vi "Client.vi"() -> ()   [LabVIEW 2015]
uses:
  <vilib>/imath/engines/lvmath2/RunTimeEngine/Managers/WorkSpace/UID Generator.vi
  <vilib>/imath/engines/lvmath/Plug In/Control Design/BuiltInFunctions/tf/NIMS_CD_tf(STR,Ts).vi
  <vilib>/imathl/engines/lvmath/Functions/Error Handling/Create Error.vi
  <vilib>/imath/engines/lvmath/Plug In/Control Design/BuiltInFunctions/multmx/NIMS_CD_multmx(TF,K).vi
  <vilib>/imath/engines/lvmath/Plug In/Control Design/BuiltInFunctions/plus/NIMS_CD_plus(K,TF).vi
  <vilib>/imath/engines/lvmath/Functions/Error Handling/MergeErrorsWrapper.vi
  <vilib>/imath/engines/lvmath/Plug In/Control Design/BuiltInFunctions/powermx/NIMS_CD_powermx(TF,N).vi
  <vilib>/imath/engines/lvmath/Plug In/Control Design/BuiltInFunctions/plus/NIMS_CD_plus(TF,TF).vi
  <vilib>/imath/engines/lvmath/Plug In/Control Design/BuiltInFunctions/rightdivmx/NIMS_CD_rightdivmx(TF,TF).vi
  <vilib>/imath/engines/lvmath2/RunTimeEngine/RunTimeType/NIMS_RunTimeType_From StrictType (excl LVString).vi
  <instcachedir>/0/NIMS_RunTimeType_From StrictType (excl LVString)_EB1C38A9BC5048DA9ABDA8F781E54D21.lvgen/NIMS_RunTimeType_From StrictType (excl LVString)_EB1C38A9BC5048DA9ABDA8F781E54D21_031.vi
  <vilib>/imath/engines/lvmath2/RunTimeEngine/LocalVariableDefStatement/MC_LocalVariableDefStatement_Display.vi
  <vilib>/imath/engines/lvmath/Plug In/Control Design/BuiltInFunctions/multmx/NIMS_CD_multmx(K,TF).vi
  <vilib>/imath/engines/lvmath/Plug In/Control Design/BuiltInFunctions/rightdivmx/NIMS_CD_rightdivmx(TF,K).vi
  <vilib>/imath/engines/lvmath/Plug In/Control Design/BuiltInFunctions/step/NIMS_CD_[Y,T]=step(TF,[Tinfo]).vi
  <vilib>/imath/engines/lvmath2/RunTimeEngine/Managers/SymbolTable/Clear UID.vi
  <vilib>/imath/engines/lvmath2/RunTimeEngine/NodeEndStatement/NIMS_NodeEndStatement_Output.vi
  <instcachedir>/0/NIMS_NodeEndStatement_Output_53EC0D466D134D7ABD903AC30B43404B.lvgen/NIMS_NodeEndStatement_Output_53EC0D466D134D7ABD903AC30B43404B_002.vi
  <vilib>/imath/engines/lvmath2/RunTimeEngine/ErrorHandling/NIMS_Finalize Error.vi
  <vilib>/imath/engines/lvmath2/RunTimeEngine/Managers/SymbolTable/NIMS_WorkSpace.lvlib
panel:
  out "JSON string":string
  in  "stop":bool
  out "error out":errorcluster
  in  "error in (no error)":errorcluster
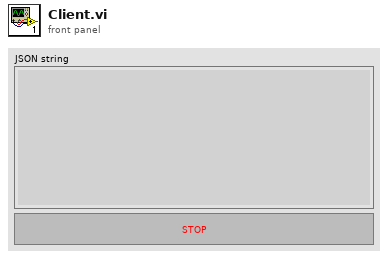
[diagram p1: front panel]
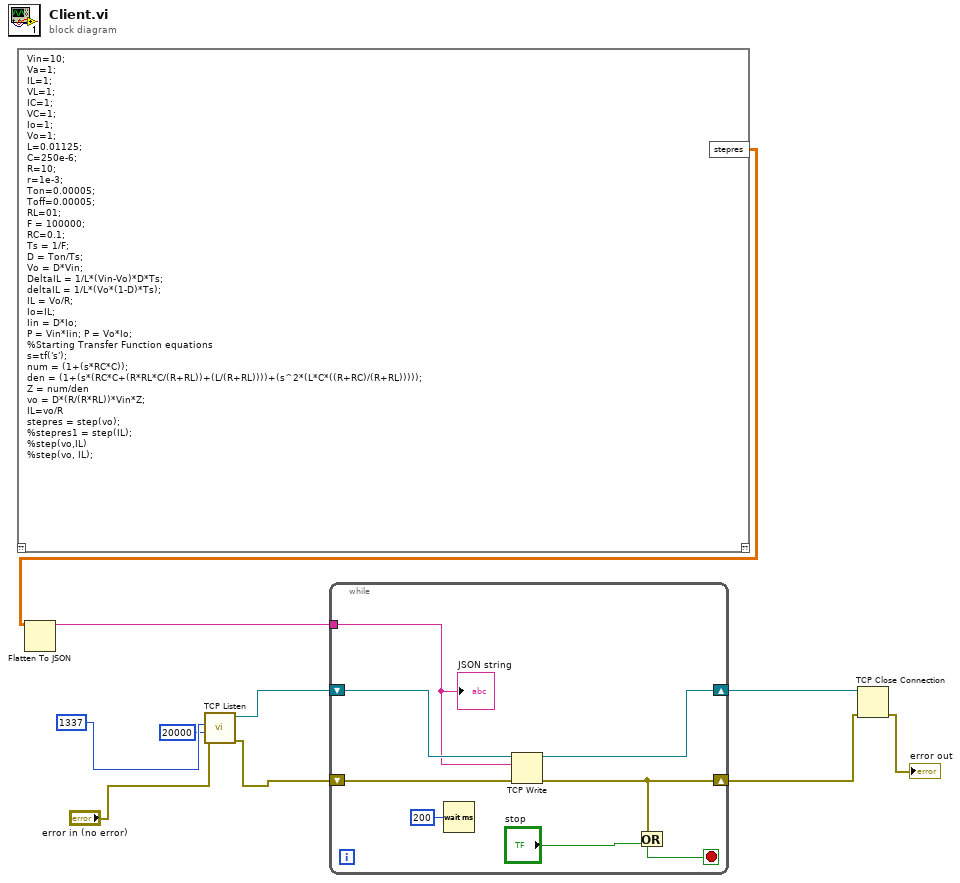
[diagram p0: block diagram]
diagram:
  n1 = mathscript code="Vin=10;\nVa=1;\nIL=1;\nVL=1;\nIC=1;\nVC=1;\nIo=1;\nVo=1;\nL=0.01125;\nC=250e-6;\nR=10;\nr=1e-3;\nTon=0.00005;\nToff=0.00005;\nRL=01;\nF = 100000;\nRC=0.1;\nTs = 1/F;\nD = Ton/Ts;\nVo = D*Vin;\nDeltaIL = 1/L*(Vin-Vo)*D*Ts;\ndeltaIL = 1/L*(Vo*(1-D)*Ts);\nIL = Vo/R;\nIo=IL;\nIin = D*Io;\nP = Vin*Iin; P = Vo*Io;\n%Starting Transfer Function equations\ns=tf('s');\nnum = (1+(s*RC*C));\nden = (1+(s*(RC*C+(R*RL*C/(R+RL))+(L/(R+RL))))+(s^2*(L*C*((R+RC)/(R+RL)))));\nZ = num/den\nvo = D*(R/(R*RL))*Vin*Z;\nIL=vo/R\nstepres = step(vo);\n%stepres1 = step(IL);\n%step(vo,IL)\n%step(vo, IL);"() -> ("stepres"=w10:dbl[][])  [unwired: 1 in, 1 out]
  n2 = Flatten To JSON(anything=w10) -> (JSON string=w9:string)  [unwired: 2 in, 1 out]
  n3 = call <vilib>:"TCP Listen.vi"("error in (no error)"="error in (no error)", "timeout ms (wait forever: -1)"=20000, "port"=1337 ("timeout ms (60000)")) -> ("error out"=w2:errorcluster, "connection ID"=w4:refnum<k5>)  [unwired: 4 in, 3 out]
  n4 = while {
    tunnel: w9 -> [w16]
    shift-right: [w15] -> w8
    shift-left: w4 -> [w18]
    shift-right: [w12] -> w7
    shift-left: w2 -> [w17]
    stop <- w14 stop-if-true
    n5 = Wait (ms)(milliseconds to wait=u32 200) -> ()  [unwired: 1 out]
    n6 = TCP Write(connection ID=w18, data in=w16, error in (no error)=w17) -> (connection ID out=w15:refnum<k5>, error out=w12:errorcluster)  [unwired: 1 in, 1 out]
    n7 = Or(x=w12, y="stop") -> (x .or. y?=w14:bool)
    "JSON string" <- w16
  }
  n8 = TCP Close Connection(connection ID=w8, error in (no error)=w7) -> (error out=→"error out":errorcluster)  [unwired: 1 in, 1 out]
